vi "特征值及向量计算.vi"() -> ()   [LabVIEW 2018]
uses:
  <vilib>/Analysis/Matrix/Datatypes/RealMatrix.ctl
  <vilib>/Analysis/7linalg.llb/Eigenvalue and Vectors Output Option.ctl
  <vilib>/Analysis/Matrix/Datatypes/ComplexMatrix.ctl
  <vilib>/Analysis/7linalg.llb/Real Eigenvalues and Vectors.vi
  <vilib>/Analysis/NI_AALPro.lvlib
  <vilib>/Analysis/Matrix/NI_Matrix.lvlib
panel:
  in  "停止":bool
  out "Eigenvectors":T1 caption="特征向量"
  out "Eigenvalues":cdb[](array[numeric]) caption="特征值"
  in  "matrix type":i32(ring) caption="矩阵类型" items=["常规", "对称"]
  in  "output option":T2=1 caption="输出选项" items=["特征值", "特征值与特征向量"]
  in  "Input Matrix":T3 caption="输入矩阵"
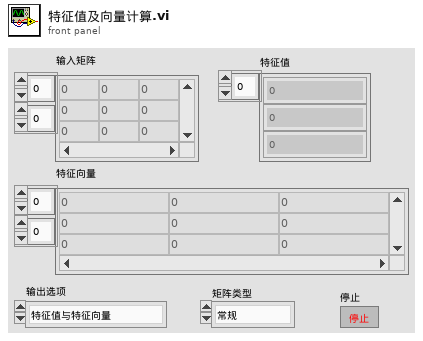
[diagram p1: front panel]
types:
  T1 = typedef "NI_Matrix.lvlib/ComplexMatrix.ctl" = cdb[][]
  T2 = typedef "NI_AALPro.lvlib/Eigenvalue and Vectors Output Option.ctl" = i32
  T3 = typedef "NI_Matrix.lvlib/RealMatrix.ctl" = dbl[][]
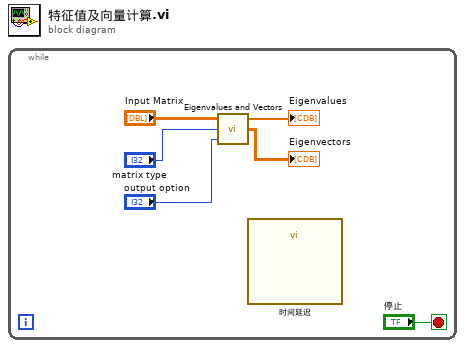
[diagram p0: block diagram]
diagram:
  n1 = while {
    stop <- "停止" stop-if-true
    n2 = call-poly <vilib>:"Eigenvalues and Vectors.vi"("output option"="output option", "matrix type"="matrix type", "Input Matrix"="Input Matrix") -> ("Eigenvectors"=→"Eigenvectors":T1, "Eigenvalues"=→"Eigenvalues":cdb[])  [unwired: 1 out]
    n3 = call "时间延迟"() -> ()  [unwired: 11 in, 1 out]
  }
